vi "SaveStabilityRecoveryFiles.vi"(2 "Arrays format":string, 3 "Array Titles":string, 7 "Sensor #":u32) -> (0 "Path + Filename OUT":string, 1 "Filename OUT":string)   [LabVIEW 2013]
uses:
  general_VIs/globals/QC_RunInformation.vi
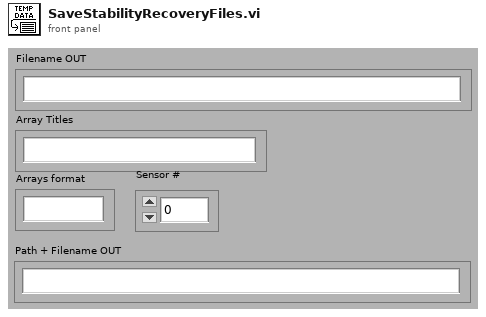
[diagram p1: front panel]
types:
  T1 = enum16{"open", "open or create", "create or replace", "create"}
  T2 = cluster{"Institute":string, "Manufacturers":string[], "Devices":string[], "Serialnumbers Lookup DB":string, "Data directory":string, "Backup & screenshot directory":string, "List of known users":string[], "Measurement switch not used":bool, "Measurement Switch":string, "DUT Switch":string, "Rseries IV [MOhm]":string, "Rshunt IV [MOhm]":string, "Rseries CV [MOhm]":string, "DC blocking Cap [µF]":string, "Rseries LCR [MOhm]":string, "Rseries stability [MOhm]":string, "Rshunt stability [MOhm]":string, "Rseries striptest bias [MOhm]":string, "Rseries strip pinhole [MOhm]":string}
  T3 = enum16{"Reset", "Read Array", "Read Element", "Write Element", "Write Array", "Add Element", "Add Array"}
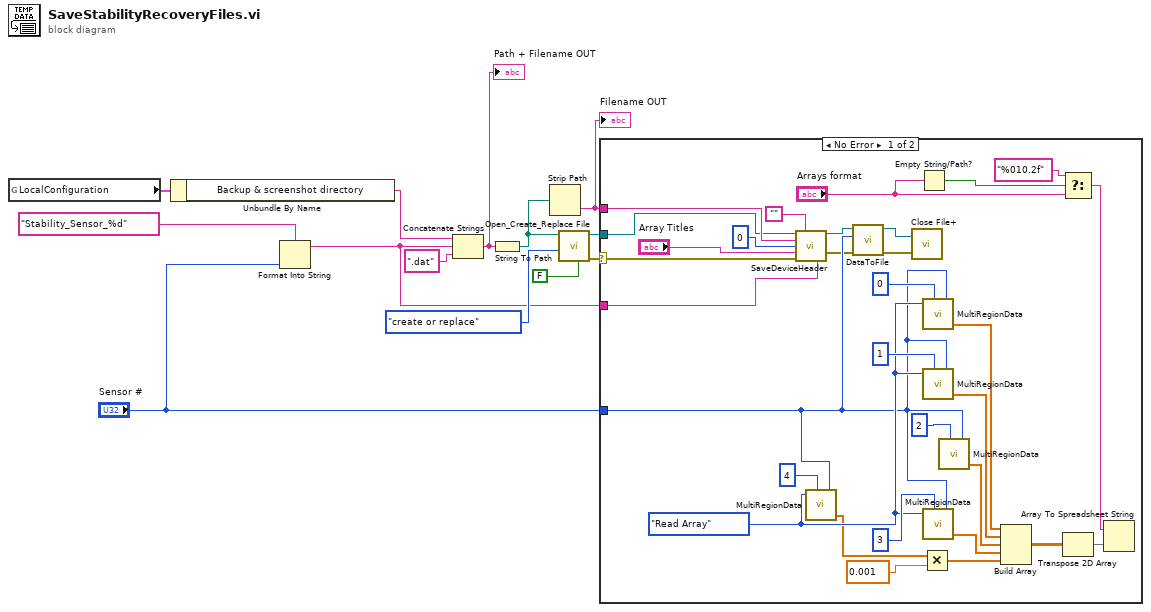
[diagram p0: block diagram]
diagram:
  n1 = global read "QC_RunInformation.vi" "LocalConfiguration"() -> (w5:T2)
  n2 = Unbundle By Name(w5) -> ("Backup & screenshot directory"=w4:string)
  n3 = Format Into String(format string="Stability_Sensor_%d", "Sensor #") -> (resulting string=w1:string)  [unwired: 2 in, 1 out]
  n4 = Concatenate Strings(w4, w1, ".dat") -> (w7:string)
  "Path + Filename OUT" <- w7
  n5 = String To Path(string=w7) -> (path=w10:path)
  n6 = Strip Path(path=w10) -> (name=w11:string)  [unwired: 1 out]
  "Filename OUT" <- w11
  n7 = call <vilib>:"Open_Create_Replace File.vi"("advisory dialog? (display:T)"=FALSE, "function (open:0)"=T1."create or replace", "file path"=w10) -> ("error out"=w9:errorcluster, "refnum"=w12:refnum<file>)  [unwired: 5 in, 2 out]
  n8 = case shown="No Error" w9 {
    selector: w9 -> [w44 _]
    tunnel: w12 -> [w41 _]
    tunnel: w11 -> [w42 _]
    tunnel: "Sensor #" -> [w19 _]
    tunnel: w1 -> [w22 _]
    frame No Error {
      w31 = T3."Read Array" ("Action")
      n9 = call "SaveDeviceHeader.vi"("File Refnum in"=w41, "Comments"="", "Filename"=w42, "Run Number"=0, "Array Titles"="Array Titles", "error in (no error)"=w44, "Strip Segment"=w22) -> ("File Refnum out"=w17:refnum<file>, "error out"=w18:errorcluster)  [unwired: 6 in, 1 out]
      n10 = call "MultiRegionData.vi"("Action"=w31, "Array No."=4, "Region index"=w19) -> ("Array OUT"=w29:dbl[])  [unwired: 3 in, 1 out]
      n11 = call "DataToFile.vi"("error in (no error)"=w18, "Sensor Index/\nSegment No."=w19, "File Refnum in"=w17) -> ("error out"=w15:errorcluster, "File Refnum out"=w16:refnum<file>)  [unwired: 7 in]
      n12 = call <vilib>:"Close File+.vi"("error in (no error)"=w15, "refnum"=w16) -> ()  [unwired: 3 in, 3 out]
      n13 = Empty String/Path?(string/path="Arrays format") -> (empty?=w40:bool)
      n14 = Multiply(x=w29, y=0.001) -> (x*y=w28:dbl[])
      n15 = call "MultiRegionData.vi"("Action"=w31, "Array No."=0, "Region index"=w19) -> ("Array OUT"=w24:dbl[])  [unwired: 3 in, 1 out]
      n16 = call "MultiRegionData.vi"("Action"=w31, "Array No."=1, "Region index"=w19) -> ("Array OUT"=w25:dbl[])  [unwired: 3 in, 1 out]
      n17 = call "MultiRegionData.vi"("Action"=w31, "Array No."=3, "Region index"=w19) -> ("Array OUT"=w27:dbl[])  [unwired: 3 in, 1 out]
      n18 = call "MultiRegionData.vi"("Array No."=2, "Region index"=w19) -> ("Array OUT"=w26:dbl[])  [unwired: 4 in, 1 out]
      n19 = Build Array(w24, w25, w26, w27, w28) -> (w23:dbl[][])
      n20 = Select(t="%010.2f", s=w40, f="Arrays format") -> (s? t:f=w37:string)
      n21 = Transpose 2D Array(2D array=w23) -> (transposed array=w14:dbl[][])
      n22 = Array To Spreadsheet String(array=w14, 3:w37) -> ()  [unwired: 1 in, 1 out]
    }
    frame Error {
    }
  }
